vi "Find Center.vi"(7 "Position":dbl format="%#_13g", 9 "XYZTheta":dbl[](array[numeric]), 11 "Gantry In":refnum<k24>) -> (1 "XYZTheta Centers":dbl[][](array[numeric]), 3 "Gantry Out":refnum<k24>)   [LabVIEW 2019, in "Pick Up Tool Fixture.lvclass"]
uses:
  Pick Up Tool Fixture.lvclass
  Controller/Camera/Machine Vision.ctl
  C:/Program Files (x86)/Aerotech/A3200/LabVIEW/2010/Bin/Aerotech.A3200.dll
  Program Files (x86)/Aerotech/A3200/LabVIEW/2010/Bin/Aerotech.A3200.dll
  Find PUT holder.ctl
  Controller/Camera/Camera.lvclass
  Controller/Motion/A3200/A3200.lvclass
panel:
  in  "BCG Values":T1={"Brightness"=128.0, "Contrast"=45.0, "Gamma"=1.0}
  in  "PUT holder":T2
  in  "Machine Vision":T3=enum."Tray Fiducials"
  out "Left Fiducial":dbl[](array[numeric])
  out "Gantry":dbl[](array[numeric])
  out "Sum":dbl[](array[numeric])
  out "Camera":dbl[](array[numeric])
  out "Image":T4(plugin-control)
  out "Center":dbl[](array[numeric])
  in  "Position Number":i16
  in  "Go to Center":bool
  in  "Calculate":bool
  in  "Record":bool
  in  "Go to Fiducial":bool
  in  "Joystick":bool
  in  "Stop":bool
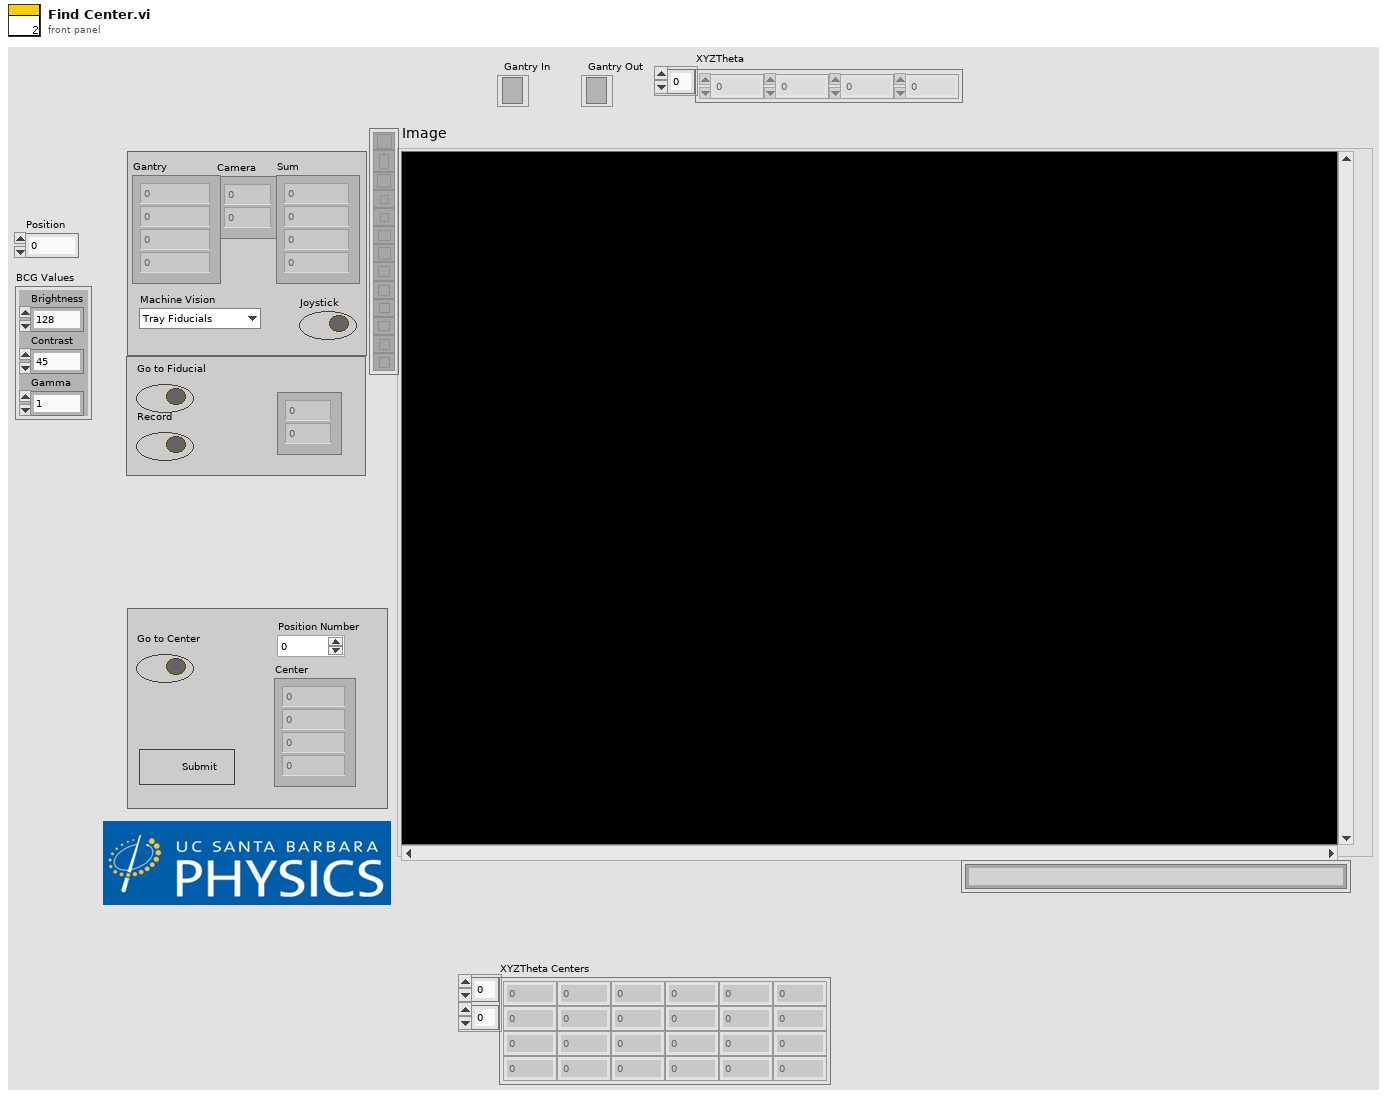
[diagram p1: front panel]
types:
  T1 = cluster{"Brightness":sgl, "Contrast":sgl, "Gamma":sgl}
  T2 = typedef "Pick Up Tool Fixture.lvclass/Find PUT holder.ctl" = cluster{"Gantry Fiducials":dbl[], "Relative Coordinates":dbl[][], "Camera Fiducials":dbl[][], "XYZTheta Centers":dbl[][], "Workspace Center":dbl[], "Gantry Region":dbl, "Fiducials":path}
  T3 = typedef "Camera.lvclass/Machine Vision.ctl" = enum16{"None", "Tray Fiducials", "HPK Silicon", "Hexaboard", "Corner (TL, BR)", "Corner (BL, TR)", "sensor TL", "sensor BL", "sensor TR", "sensor BR", "hexaboard TL", "hexaboard BL", "hexaboard TR", "hexaboard BR"}
  T4 = typedef "IMAQ Image.ctl" = refnum<image>
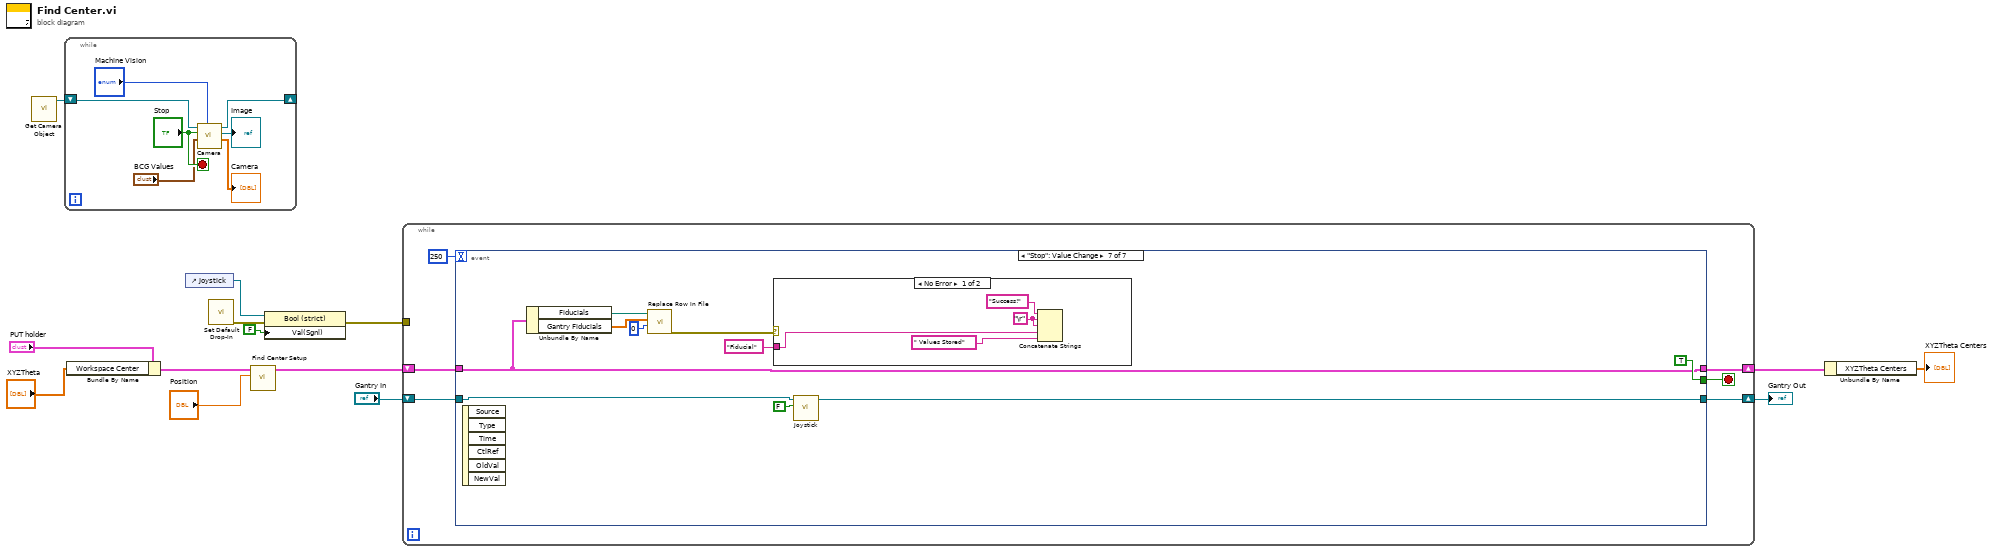
[diagram p0: block diagram]
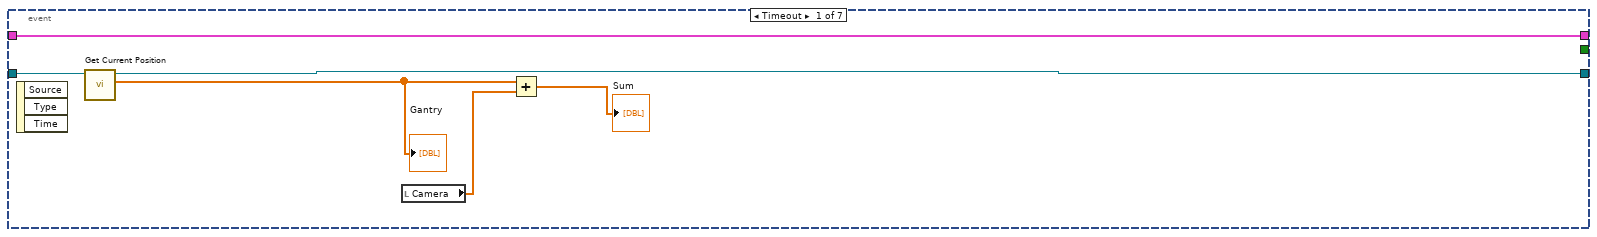
[diagram p2: hidden frame]
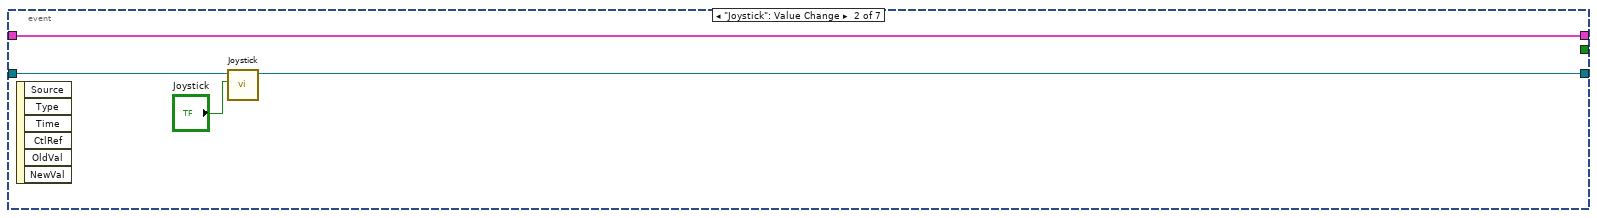
[diagram p3: hidden frame]
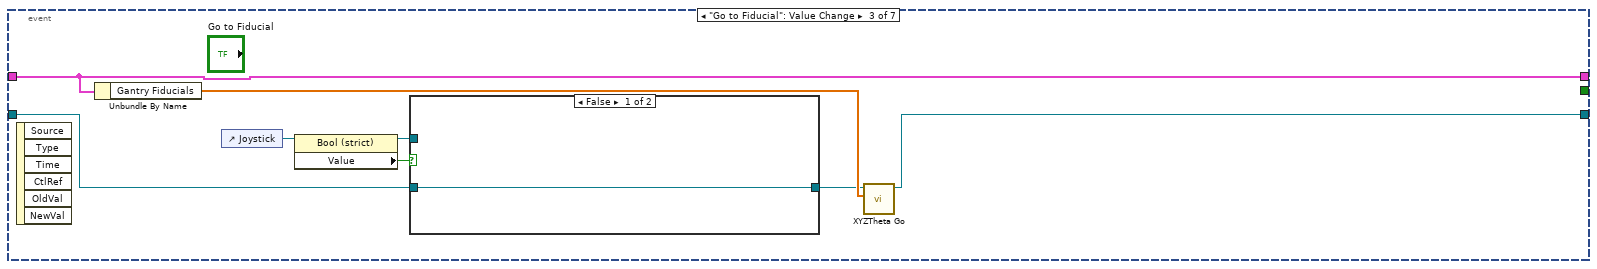
[diagram p4: hidden frame]
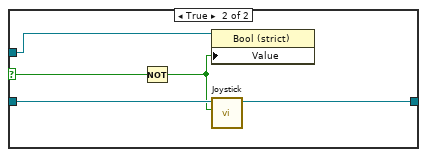
[diagram p5: hidden frame]
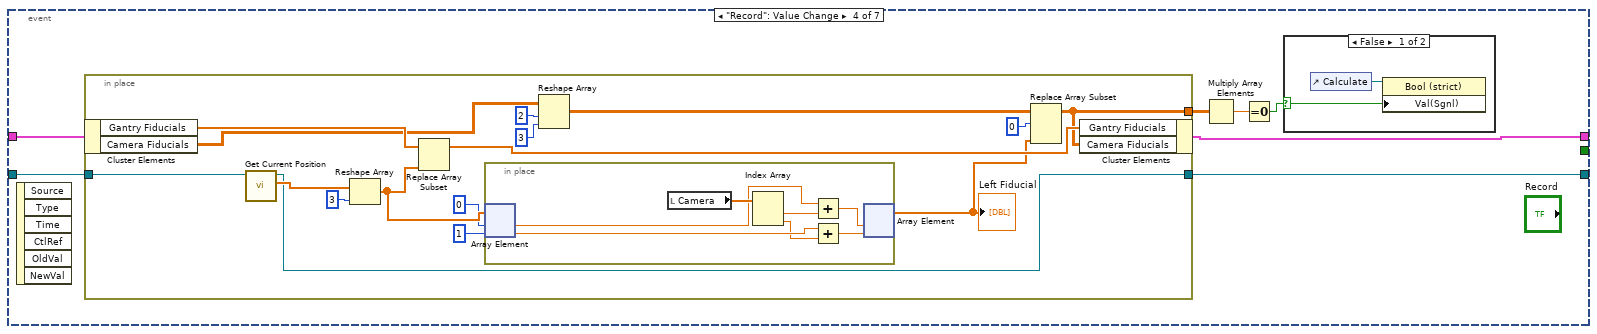
[diagram p6: hidden frame]
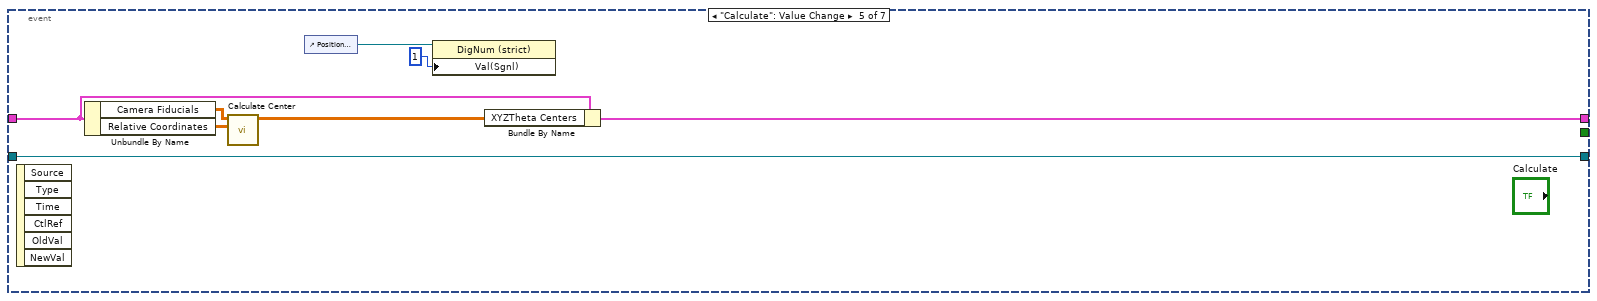
[diagram p8: hidden frame]
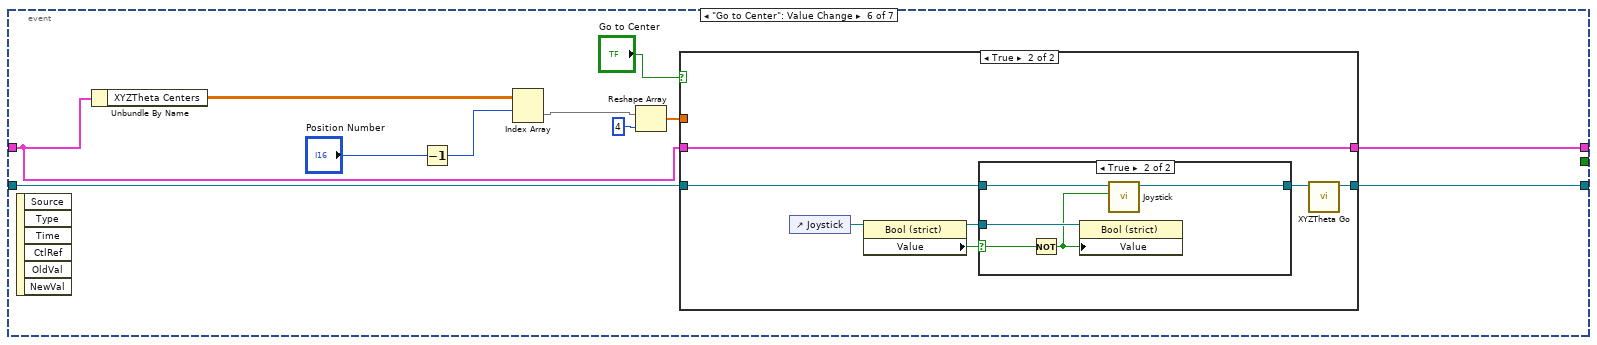
[diagram p9: hidden frame]
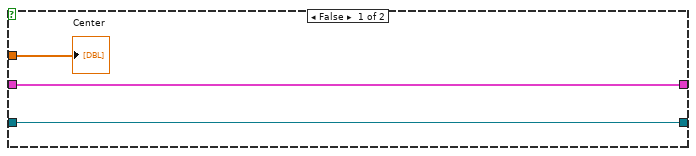
[diagram p10: hidden frame]
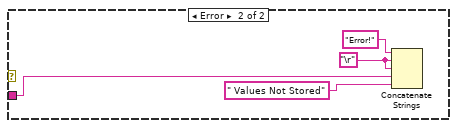
[diagram p12: hidden frame]
diagram:
  n1 = call "Get Camera Object.vi"() -> ("Camera out"=w14:refnum<class "Camera.lvclass">)  [unwired: 10 in, 1 out]
  n2 = while {
    shift-right: [w19] -> _
    shift-left: w14 -> [w20]
    stop <- "Stop" stop-if-true
    n3 = call "Camera.vi"("Machine Vision"="Machine Vision", "BCG Values"="BCG Values", "Stop"="Stop", "Camera in"=w20) -> ("Camera"=→"Camera":dbl[], "Image"=→"Image":T4, "Camera out"=w19:refnum<class "Camera.lvclass">)  [unwired: 4 in, 1 out]
  }
  n4 = Bundle By Name(cluster="PUT holder", "Workspace Center"="XYZTheta") -> (w9:T2)
  n5 = control-ref of="Joystick"() -> (w6:refnum<vi>)
  n6 = call "Set Default Drop-In.vi"() -> ("error out"=w5:errorcluster)  [unwired: 11 in]
  n7 = call "Find Center Setup.vi"("Position"="Position", "PUT holder in"=w9) -> ("PUT holder out"=w7:T2)  [unwired: 9 in]
  n8 = property class="Bool (strict)"(reference=w6, error in=w5, "Val(Sgnl)"=FALSE ("Value (Signaling)")) -> (error out=w3:errorcluster)  [unwired: 1 out]
  n9 = while {
    shift-right: [w26] -> w12
    shift-left: "Gantry In" -> [w27]
    shift-right: [w23] -> w1
    shift-left: w7 -> [w24]
    tunnel: w3 -> [_]
    stop <- w25 stop-if-true
    n10 = event shown="[6] \"Stop\": Value Change" {
      selector: _ -> [_ _ _ _ _ _ _]
      dyn-events: _ -> [_ _ _ _ _ _ _]
      timeout: 250 -> [_ _ _ _ _ _ _]
      tunnel: w27 -> [w33 w37 w39 w57 w86 w95 w124]
      tunnel: [w32 w35 w43 w52 w86 w94 w122] -> w26
      tunnel: [_ _ _ _ _ _ TRUE] -> w25
      tunnel: w24 -> [w28 w34 w45 w58 w88 w92 w121]
      tunnel: [w28 w34 w45 w53 w87 w93 w121] -> w23
      event Timeout {
        n11 = event-data() -> ()  [unwired: 1 in, 3 out]
        n12 = call "Get Current Position.vi"("Gantry In"=w33) -> ("XYZTheta Out"=w31:dbl[], "Gantry Out"=w32:refnum<k24>)  [unwired: 8 in, 1 out]
        "Gantry" <- w31
        n13 = local read "Camera"() -> (w29:dbl[])
        n14 = Add(x=w31, y=w29) -> (x+y=→"Sum":dbl[])
      }
      event "Joystick": Value Change {
        n15 = event-data() -> ()  [unwired: 1 in, 6 out]
        n16 = call "Joystick.vi"("Joystick"="Joystick", "Gantry In"=w37) -> ("Gantry Out"=w35:refnum<k24>)  [unwired: 8 in, 1 out]
      }
      event "Go to Fiducial": Value Change {
        n17 = event-data() -> ()  [unwired: 1 in, 6 out]
        n18 = Unbundle By Name(w45) -> ("Gantry Fiducials"=w44:dbl[])
        n19 = control-ref of="Joystick"() -> (w42:refnum<vi>)
        n20 = property class="Bool (strict)"(reference=w42) -> (reference out=w41:refnum<vi>, "Value"=w40:bool)  [unwired: 1 in, 1 out]
        n21 = case shown="False" w40 {
          selector: w40 -> [_ w51]
          tunnel: w39 -> [w46 w49]
          tunnel: [w46 w48] -> w38
          tunnel: w41 -> [_ w50]
          frame False {
          }
          frame True {
            n22 = Not(x=w51) -> (.not. x?=w47:bool)
            n23 = property class="Bool (strict)"(reference=w50, "Value"=w47) -> ()  [unwired: 1 in, 2 out]
            n24 = call "Joystick.vi"("Joystick"=w47, "Gantry In"=w49) -> ("Gantry Out"=w48:refnum<k24>)  [unwired: 8 in, 1 out]
          }
        }
        n25 = call "XYZTheta Go.vi"("XYZTheta In"=w44, "Gantry In"=w38) -> ("Gantry Out"=w43:refnum<k24>)  [unwired: 7 in, 2 out]
      }
      event "Record": Value Change {
        n26 = event-data() -> ()  [unwired: 1 in, 6 out]
        n27 = in-place {
          in-place-border: w57 -> [w76]
          in-place-border: [w62] -> w55
          in-place-border: [w61] -> w52
          n28 = in-place-cluster #1(w58) -> ("Gantry Fiducials"=w75:dbl[], "Camera Fiducials"=w72:dbl[][])
          n29 = call "Get Current Position.vi"("Gantry In"=w76) -> ("XYZTheta Out"=w74:dbl[], "Gantry Out"=w61:refnum<k24>)  [unwired: 8 in, 1 out]
          n30 = Reshape Array(w74, 3 ("dimension size")) -> (w67:dbl[])
          n31 = Replace Array Subset(array=w75, new element=w67) -> (w66:dbl[])  [unwired: 1 in]
          n32 = in-place {
            n33 = in-place-array #2(w67, 0, 1) -> (w81:dbl, w80:dbl)
            n34 = local read "Camera"() -> (w83:dbl[])
            n35 = Index Array(array=w83) -> (element #1=w82:dbl, element #2=w79:dbl)  [unwired: 2 in]
            n36 = Add(x=w81, y=w82) -> (x+y=w78:dbl)
            n37 = Add(x=w80, y=w79) -> (x+y=w77:dbl)
            n38 = in-place-array #2(w78, w77) -> (w63:dbl[])  [unwired: 2 out]
          }
          "Left Fiducial" <- w63
          n39 = Reshape Array(w72, 2 ("dimension size"), 3 ("dimension size")) -> (w69:dbl[][])
          n40 = Replace Array Subset(array=w69, new element=w63, index (row)=0) -> (w62:dbl[][])  [unwired: 1 in]
          n41 = in-place-cluster #1("Gantry Fiducials"=w66, "Camera Fiducials"=w62) -> (w53:T2)
        }
        n42 = Multiply Array Elements(1:w55) -> (0:w56:dbl)
        n43 = Equal To 0?(x=w56) -> (x = 0?=w54:bool)
        n44 = case shown="False" w54 {
          selector: w54 -> [w59 _]
          frame False {
            n45 = control-ref of="Calculate"() -> (w60:refnum<vi>)
            n46 = property class="Bool (strict)"(reference=w60, "Val(Sgnl)"=w59) -> ()  [unwired: 1 in, 2 out]
          }
          frame True {
          }
        }
      }
      event "Calculate": Value Change {
        n47 = event-data() -> ()  [unwired: 1 in, 6 out]
        n48 = Unbundle By Name(w88) -> ("Camera Fiducials"=w91:dbl[][], "Relative Coordinates"=w90:dbl[][])
        n49 = call "Calculate Center.vi"("Relative Coordinates"=w90, "Fiducial Measurements"=w91) -> ("XYZTheta Centers"=w89:dbl[][])  [unwired: 9 in]
        n50 = control-ref of="Position Number"() -> (w85:refnum<vi>)
        n51 = property class="DigNum (strict)"(reference=w85, "Val(Sgnl)"=i16 1 ("Value (Signaling)")) -> ()  [unwired: 1 in, 2 out]
        n52 = Bundle By Name(cluster=w88, "XYZTheta Centers"=w89) -> (w87:T2)
      }
      event "Go to Center": Value Change {
        n53 = event-data() -> ()  [unwired: 1 in, 6 out]
        n54 = Unbundle By Name(w92) -> ("XYZTheta Centers"=w101:dbl[][])
        n55 = Decrement(x="Position Number") -> (x-1=w100:i16)
        n56 = Index Array(array=w101, index (row)=w100) -> (element=w99:dbl[])  [unwired: 1 in]
        n57 = Reshape Array(w99, 4 ("dimension size")) -> (w96:dbl[])
        n58 = case shown="True" "Go to Center" {
          tunnel: w96 -> [w105 _]
          tunnel: w95 -> [w103 w108]
          tunnel: [w103 w106] -> w94
          tunnel: [w104 w112] -> w93
          tunnel: w92 -> [w104 w112]
          frame False {
            "Center" <- w105
          }
          frame True {
            n59 = control-ref of="Joystick"() -> (w111:refnum<vi>)
            n60 = property class="Bool (strict)"(reference=w111) -> (reference out=w109:refnum<vi>, "Value"=w110:bool)  [unwired: 1 in, 1 out]
            n61 = case shown="True" w110 {
              selector: w110 -> [_ w118]
              tunnel: w109 -> [_ w117]
              tunnel: w108 -> [w113 w116]
              tunnel: [w113 w115] -> w107
              frame False {
              }
              frame True {
                n62 = Not(x=w118) -> (.not. x?=w114:bool)
                n63 = property class="Bool (strict)"(reference=w117, "Value"=w114) -> ()  [unwired: 1 in, 2 out]
                n64 = call "Joystick.vi"("Joystick"=w114, "Gantry In"=w116) -> ("Gantry Out"=w115:refnum<k24>)  [unwired: 8 in, 1 out]
              }
            }
            n65 = call "XYZTheta Go.vi"("Gantry In"=w107) -> ("Gantry Out"=w106:refnum<k24>)  [unwired: 8 in, 2 out]
          }
        }
      }
      event "Stop": Value Change {
        n66 = event-data() -> ()  [unwired: 1 in, 6 out]
        n67 = Unbundle By Name(w121) -> ("Fiducials"=w127:path, "Gantry Fiducials"=w126:dbl[])
        n68 = call "Replace Row In File.vi"("Index"=0, "Insert Array"=w126, "Path"=w127) -> ("error out"=w120:errorcluster)  [unwired: 8 in]
        n69 = case shown="No Error" w120 {
          tunnel: "Fiducial" -> [w129 w136]
          frame No Error {
            w130 = "\r"
            n70 = Concatenate Strings("Success!", w130, w130, w129, " Values Stored") -> ()  [unwired: 1 out]
          }
          frame Error {
            w133 = "\r"
            n71 = Concatenate Strings("Error!", w133, w133, w136, " Values Not Stored") -> ()  [unwired: 1 out]
          }
        }
        n72 = call "Joystick.vi"("Joystick"=FALSE, "Gantry In"=w124) -> ("Gantry Out"=w122:refnum<k24>)  [unwired: 8 in, 1 out]
      }
    }
  }
  "Gantry Out" <- w12
  n73 = Unbundle By Name(w1) -> ("XYZTheta Centers"=→"XYZTheta Centers":dbl[][])
